vi "frw_decode_header.vi"(10 "header2":string, 11 "header1":string) -> (0 "tags":string, 1 "live?":bool, 2 "chLabels":string, 3 "header1 out":string, 4 "fs":i32, 6 "hardware":string)   [LabVIEW 2013]
doc: "Decodes the CSV header to get information about the recording"
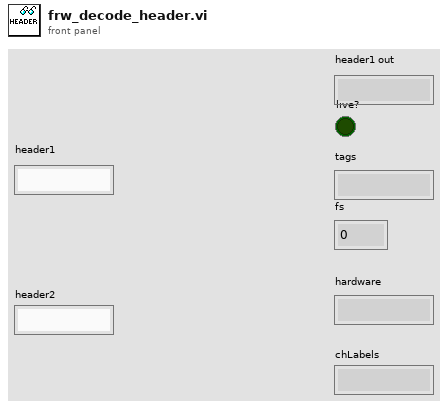
[diagram p1: front panel]
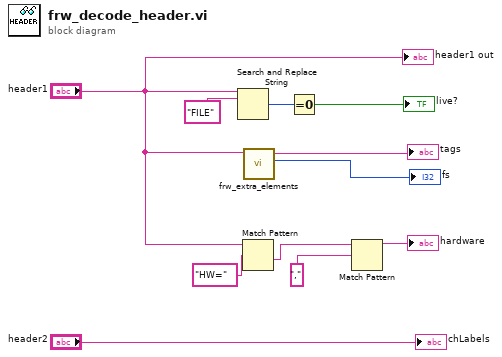
[diagram p0: block diagram]
diagram:
  n1 = Search and Replace String(input string="header1", search string="FILE" ("string")) -> (number of replacements=w11:i32)  [unwired: 6 in, 3 out]
  n2 = Match Pattern(string="header1", regular expression="HW=" ("delimiter (Tab)")) -> (after substring=w5:string)  [unwired: 1 in, 3 out]
  n3 = call "frw_extra_elements.vi"("string"="header1") -> ("fs"=→"fs":i32, "data_format"=→"tags":string)  [unwired: 6 in, 3 out]
  n4 = Equal To 0?(x=w11) -> (x = 0?=→"live?":bool)
  n5 = Match Pattern(string=w5, regular expression="," ("delimiter (Tab)")) -> (before substring=→"hardware":string)  [unwired: 1 in, 3 out]
  "chLabels" <- "header2"
  "header1 out" <- "header1"
